vi "CheckLoopLF.vi"(11 "Code":string) -> (3 "Code fixed":string)   [LabVIEW 2016]
panel:
  out "Array":string[](array[string])
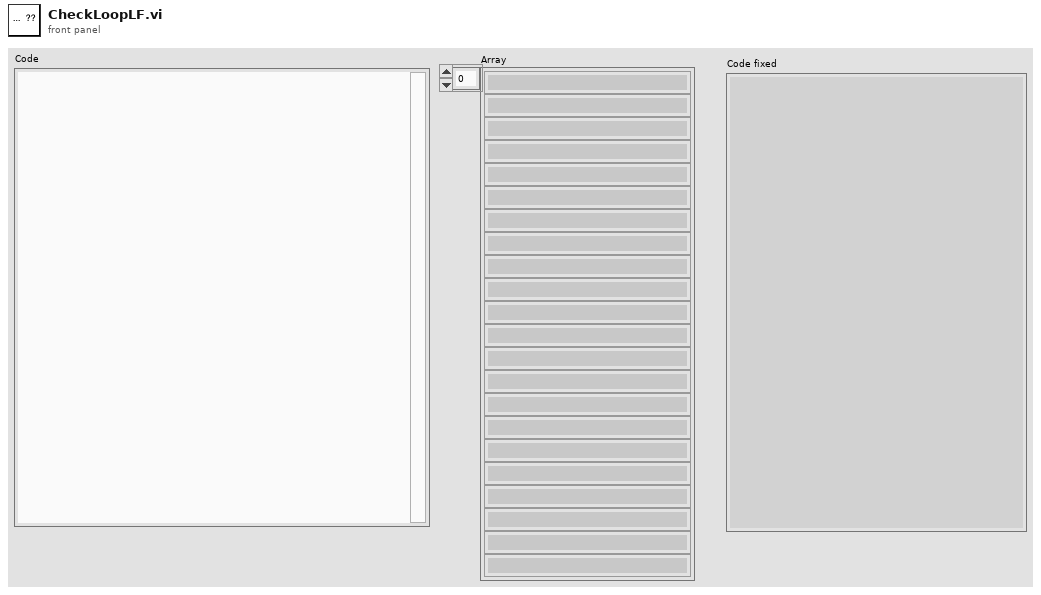
[diagram p1: front panel]
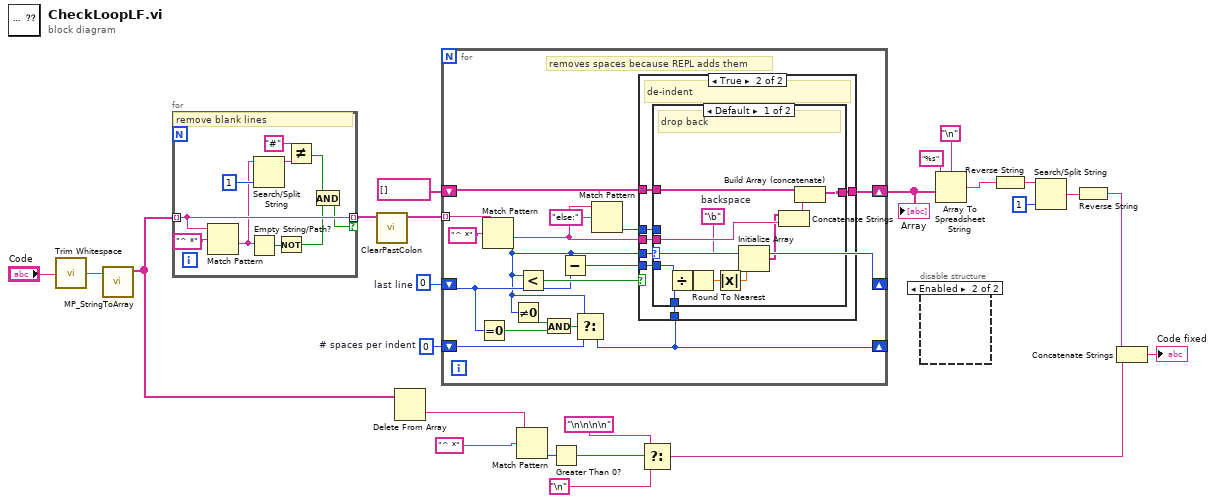
[diagram p0: block diagram]
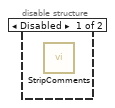
[diagram p2: hidden frame]
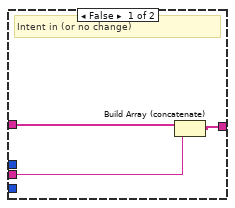
[diagram p3: hidden frame]
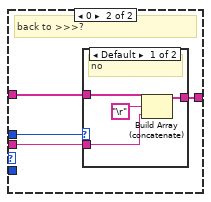
[diagram p4: hidden frame]
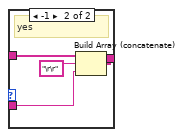
[diagram p5: hidden frame]
diagram:
  w1 = 0  # # spaces per indent
  w16 = 0  # last line
  n1 = call <vilib>:"Trim Whitespace.vi"("string"="Code") -> ("trimmed string"=w13:string)  [unwired: 1 in]
  n2 = call "MP_StringToArray.vi"("write buffer"=w13) -> ("Array"=w4:string[])  [unwired: 10 in]
  n3 = for {
    tunnel: w4 -> [w33] mode=indexing
    tunnel: [w33] -> w3 mode=indexing if=w25
    # "remove blank lines"
    n4 = Match Pattern(string=w33, regular expression="^ *") -> (after substring=w30:string)  [unwired: 1 in, 3 out]
    n5 = Empty String/Path?(string/path=w30) -> (empty?=w32:bool)
    n6 = Search/Split String(string=w30, offset (0)=1) -> (substring before match=w29:string)  [unwired: 1 in, 2 out]
    n7 = Not(x=w32) -> (.not. x?=w26:bool)
    n8 = Not Equal?(x="#", y=w29) -> (x != y?=w27:bool)
    n9 = And(x=w27, y=w26) -> (x .and. y?=w25:bool)
  }
  n10 = call "ClearPastColon.vi"("Array in"=w3) -> ("Array out"=w2:string[])  [unwired: 10 in]
  n11 = Delete From Array(array=w4) -> (deleted portion=w20:string)  [unwired: 2 in, 1 out]
  n12 = for {
    tunnel: w2 -> [w47] mode=indexing
    shift-right: [w35] -> _
    shift-left: w16 -> [w38]
    shift-right: [w46] -> w14
    shift-left: string[] [] ("Array") -> [w48]
    shift-right: [w36] -> _
    shift-left: w1 -> [w39]
    # "removes spaces because REPL adds them"
    n13 = Equal To 0?(x=w38) -> (x = 0?=w42:bool)
    n14 = Match Pattern(string=w47, regular expression="^ *") -> (after substring=w45:string, offset past match=w35:i32)  [unwired: 1 in, 2 out]
    n15 = Not Equal To 0?(x=w35) -> (x != 0?=w41:bool)
    n16 = Less?(x=w35, y=w38) -> (x < y?=w49:bool)
    n17 = And(x=w41, y=w42) -> (x .and. y?=w40:bool)
    n18 = Subtract(x=w35, y=w38) -> (x-y=w37:i32)
    n19 = Select(t=w35, s=w40, f=w39) -> (s? t:f=w36:i32)
    n20 = Match Pattern(string=w45, regular expression="else:") -> (offset past match=w43:i32)  [unwired: 1 in, 3 out]
    n21 = case shown="True" w49 {
      tunnel: w48 -> [w53 w60]
      tunnel: w45 -> [w52 w58]
      tunnel: [w51 w59] -> w46
      tunnel: w35 -> [_ w57]
      tunnel: w43 -> [_ w56]
      tunnel: w37 -> [_ w55]
      tunnel: w36 -> [_ w54]
      frame False {
        # "Intent in (or no change)"
        n22 = Build Array (concatenate)(w53, w52) -> (w51:string[])
      }
      frame True {
        # "de-indent"
        n23 = case shown="Default" w57 {
          tunnel: w60 -> [w71 w75]
          tunnel: [w70 w74] -> w59
          tunnel: w58 -> [w69 w73]
          tunnel: w56 -> [_ w72]
          tunnel: w55 -> [w64 _]
          tunnel: w54 -> [w63 _]
          frame Default {
            w67 = "\b"  # backspace
            # "drop back"
            n24 = Divide(x=w64, y=w63) -> (x/y=w62:dbl)
            n25 = Round To Nearest(number=w62) -> (nearest integer value=w61:dbl)
            n26 = Absolute Value(x=w61) -> (abs(x)=w65:dbl)
            n27 = Initialize Array(w67, w65) -> (w66:string[])
            n28 = Concatenate Strings(w66, w69) -> (w68:string)
            n29 = Build Array (concatenate)(w71, w68) -> (w70:string[])
          }
          frame 0 {
            # "back to >>>?"
            n30 = case shown="Default" w72 {
              tunnel: w75 -> [w78 w83]
              tunnel: [w77 w82] -> w74
              tunnel: w73 -> [w76 w81]
              frame Default {
                # "no"
                n31 = Build Array (concatenate)(w78, "\r" ("regular expression"), w76) -> (w77:string[])
              }
              frame -1 {
                # "yes"
                n32 = Build Array (concatenate)(w83, "\r\r" ("regular expression"), w81) -> (w82:string[])
              }
            }
          }
        }
      }
    }
  }
  "Array" <- w14
  n33 = Match Pattern(string=w20, regular expression="^ *") -> (offset past match=w22:i32)  [unwired: 1 in, 3 out]
  n34 = Greater Than 0?(x=w22) -> (x > 0?=w21:bool)
  n35 = Select(t="\n\n\n\n", s=w21, f="\n") -> (s? t:f=w17:string)
  n36 = disable-structure shown="Enabled" {
    frame Disabled {
      n37 = call "StripComments.vi"() -> ()  [unwired: 10 in, 2 out]
    }
    frame Enabled {
    }
  }
  n38 = Array To Spreadsheet String(delimiter (Tab)="\n", array=w14, 3:"%s" ("format string")) -> (spreadsheet string=w9:string)
  n39 = Reverse String(1:w9) -> (0:w8:string)
  n40 = Search/Split String(string=w8, offset (0)=1) -> (match + rest of string=w6:string)  [unwired: 1 in, 2 out]
  n41 = Reverse String(1:w6) -> (0:w5:string)
  n42 = Concatenate Strings(w5, w17) -> (→"Code fixed":string)
